vi "Extract TSM DAQmx Multiple SSC.vi"(0 "DAQmx Tasks":refnum<k21>[](array[refnum]), 5 "Channel Lists":string[](array[string]), 7 "Per-Session Channel List":string[](array[string])) -> (4 "DAQ TSM SSC Multiple Out":T1[](array[typedef]))   [LabVIEW 2019]
uses:
  DAQmx/Pin Map/SSC DAQmx.ctl
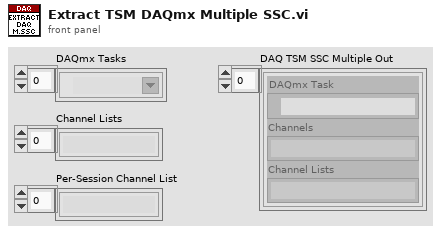
[diagram p1: front panel]
types:
  T1 = typedef "SSC DAQmx.ctl" = cluster{"DAQmx Task ":refnum<k21>, "Channels":string, "Channel Lists":string}
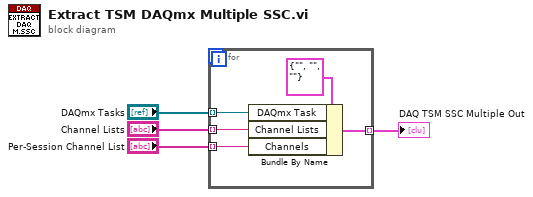
[diagram p0: block diagram]
diagram:
  n1 = for {
    tunnel: "DAQmx Tasks" -> [w8] mode=indexing
    tunnel: "Channel Lists" -> [w7] mode=indexing
    tunnel: "Per-Session Channel List" -> [w6] mode=indexing
    tunnel: [w5] -> w4 mode=indexing
    n2 = Bundle By Name(cluster=T1 {"DAQmx Task "="", "Channels"="", "Channel Lists"=""} ("DAQmx SSC"), "DAQmx Task"=w8, "Channel Lists"=w7, "Channels"=w6) -> (w5:T1)
  }
  "DAQ TSM SSC Multiple Out" <- w4
